vi "FPGA Main.vi"() -> ()   [LabVIEW 2021]
uses:
  <vilib>/Platform/TimedLoop/XDataNode/timing_clust.ctl
  <vilib>/Platform/TimedLoop/XDataNode/nitl_modes.ctl
  <vilib>/Platform/TimedLoop/XDataNode/wakeup.ctl
  <vilib>/rvi/Emulation/niFpgaSctlEmulationGetInTimedLoop.vi
  <vilib>/rvi/Emulation/niFpgaEmulationReportErrorSimple.vi
  <vilib>/rvi/Emulation/niFpgaGetClockAttributes.vi
  <vilib>/rvi/Emulation/niFpgaCriticalErrorInLSC.vi
  <vilib>/rvi/eio/common/nirviEmuTemplateMethod_errors.vi
  <vilib>/rvi/interface/RandomDataEmulation/niFpgaRandomDataHandleErrors.vi
  <vilib>/platform/TimedLoop/XDataNode/XDataNode.xnode
  <vilib>/eio/EIONode/EIONode.xnode
  <vilib>/rvi/DataTransferAndStorage/Container/XNode/niFpgaContainer.xnode
  <vilib>/rvi/interface/RandomDataEmulation/nirviRandomDataFpgaReadWriteTemplate.vi
  <vilib>/Platform/TimedLoop/XDataNode/XDNodeRunTimeDep.lvlib
panel:
  in  "Count(uSec)":u32
  out "Overflow?":bool
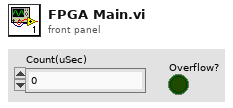
[diagram p1: front panel]
types:
  T1 = typedef "XDNodeRunTimeDep.lvlib/timing_clust.ctl" = cluster{"Expected End [f-1]":u64, "Actual End [f-1]":u64, "Finished Late? [f-1]":bool, "Expected End [i-1]":u64, "Actual End [i-1]":u64, "Finished Late? [i-1]":bool, "Expected Start [i]":u64, "Actual Start [i]":u64, "Expected Start [f]":u64, "Actual Start [f]":u64, "Source Name":string, "Structure Name":string, "Period":i64, "Deadline":i64, "Offset":i64, "Start":i64, "Priority":i32, "Timeout":i32, "Mode":T2, "Wakeup Reason":T3, "Error":errorcluster, "Source Type":string, "Secondary Source Type":string, "Global End Time":u64, "Global Start Time":u64, "Frame Duration":u64, "Iteration Duration":u64, "Assigned CPU":i32, "I/O Scan Engine Mode":u32}
  T2 = typedef "XDNodeRunTimeDep.lvlib/nitl_modes.ctl" = enum32{"No Change", "Process missed periods, maintain original phase", "Discard missed periods, maintain original phase", "Process missed periods, ignore original phase", "Discard missed periods, ignore original phase"}
  T3 = typedef "XDNodeRunTimeDep.lvlib/wakeup.ctl" = enum32{"Normal", "Aborted", "Asynchronous wakeup", "Timing source error", "Timed loop error", "Timeout"}
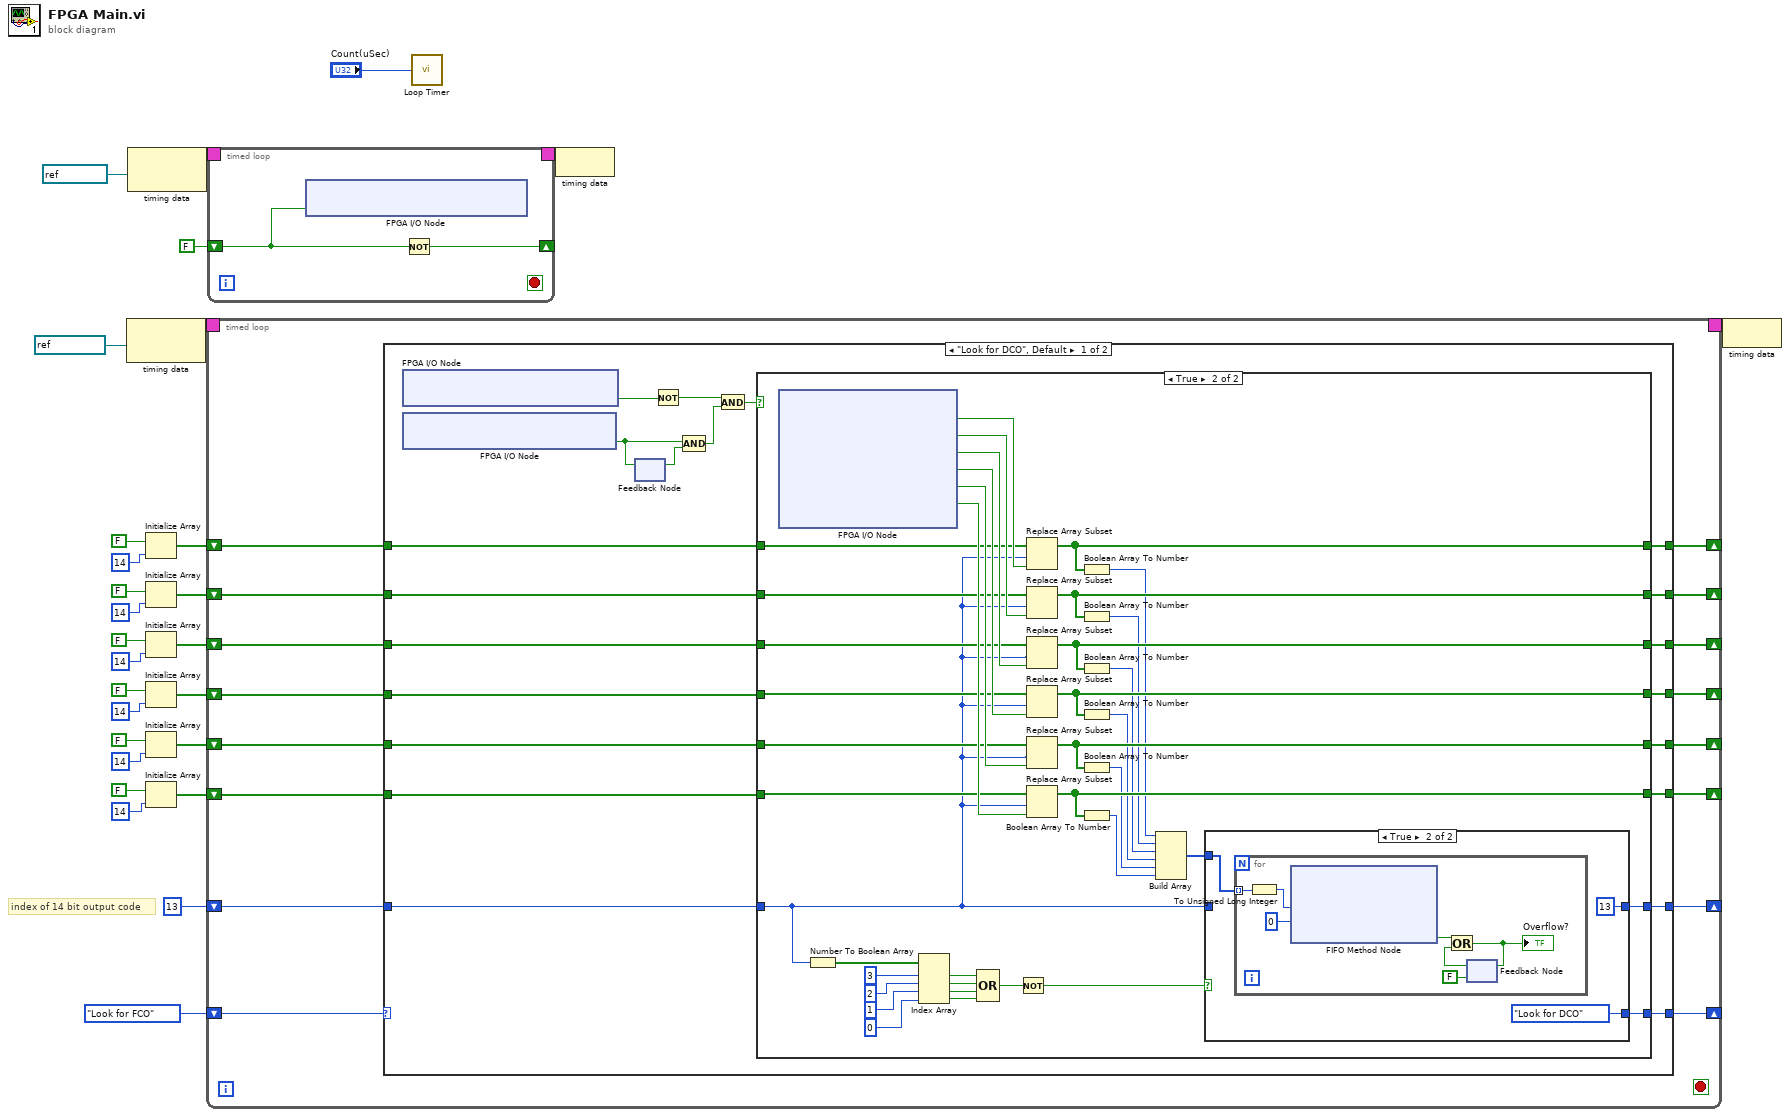
[diagram p0: block diagram]
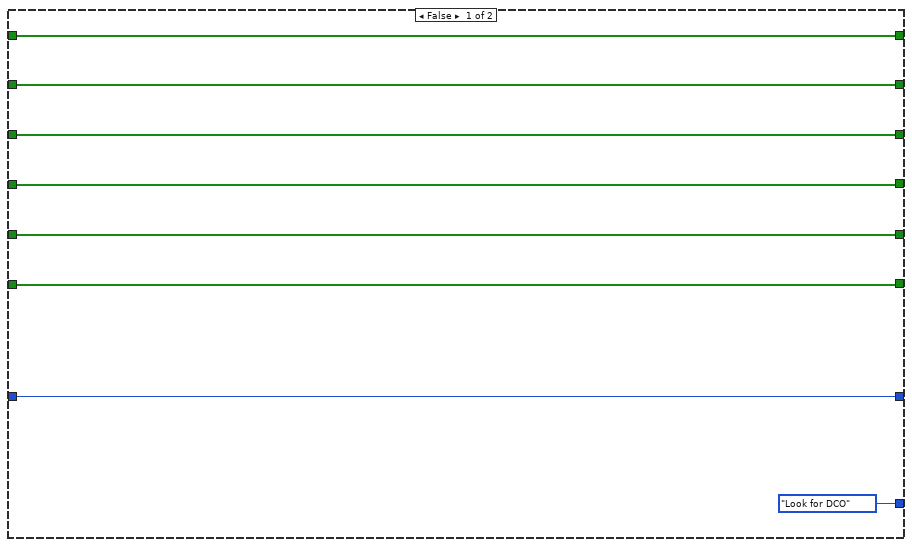
[diagram p2: hidden frame]
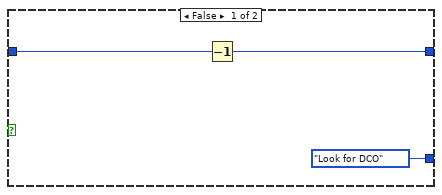
[diagram p3: hidden frame]
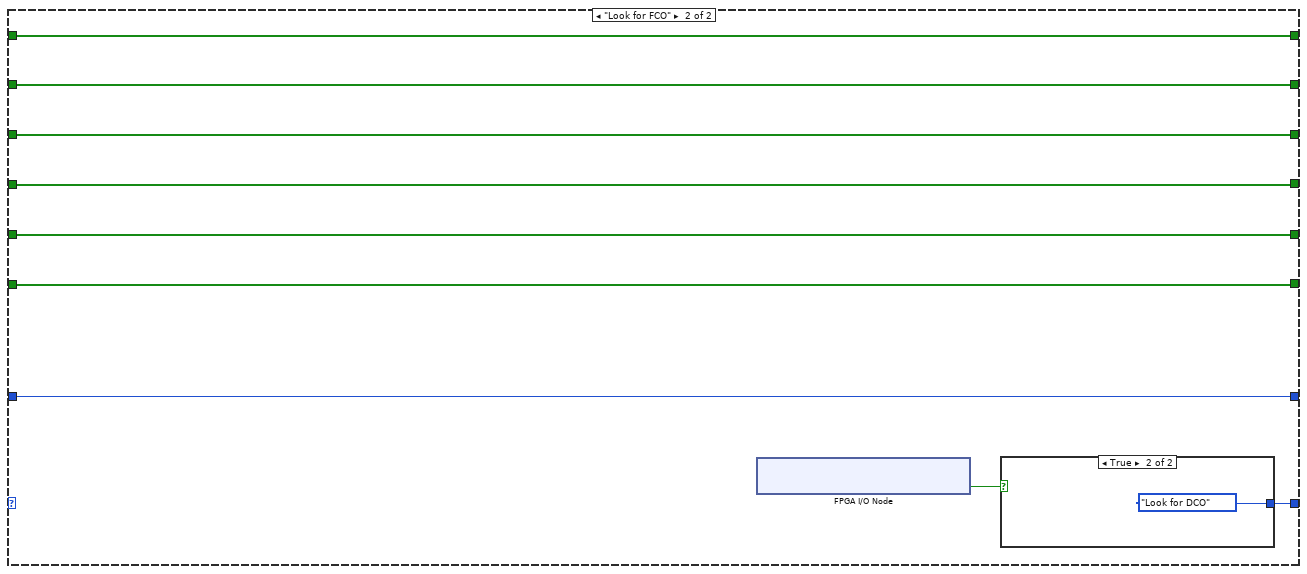
[diagram p4: hidden frame]
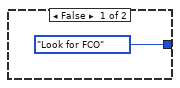
[diagram p5: hidden frame]
diagram:
  # "index of 14 bit output code"
  n1 = node-c288(refnum<k21> "140MHz" ("Source Name")) -> (w24:T1)
  n2 = node-c288(refnum<k21> "20MHz" ("Source Name")) -> (w28:T1)
  n3 = Initialize Array(FALSE, 14) -> (w7:bool[])
  n4 = Initialize Array(FALSE, 14) -> (w6:bool[])
  n5 = Initialize Array(FALSE, 14) -> (w5:bool[])
  n6 = Initialize Array(FALSE, 14) -> (w4:bool[])
  n7 = Initialize Array(FALSE, 14) -> (w3:bool[])
  n8 = Initialize Array(FALSE, 14) -> (w2:bool[])
  n9 = timed-loop {
    timing: w24 -> [_]
    timing-out: [_] -> w23
    shift-right: [w43] -> _
    shift-left: 13 ("index") -> [w44]
    shift-right: [w41] -> _
    shift-left: enum16{"Look for DCO", "Look for FCO"}."Look for FCO" -> [w42]
    shift-right: [w34] -> _
    shift-left: w7 -> [w40]
    shift-right: [w33] -> _
    shift-left: w6 -> [w39]
    shift-right: [w32] -> _
    shift-left: w5 -> [w38]
    shift-right: [w31] -> _
    shift-left: w4 -> [w37]
    shift-right: [w30] -> _
    shift-left: w3 -> [w36]
    shift-right: [w29] -> _
    shift-left: w2 -> [w35]
    stop <- _ stop-if-true
    n10 = case shown="\"Look for DCO\", Default" w42 {
      tunnel: w44 -> [w65 w132]
      tunnel: [w64 w132] -> w43
      tunnel: [w61 w134] -> w41
      tunnel: w40 -> [w56 w131]
      tunnel: w39 -> [w55 w130]
      tunnel: w38 -> [w54 w129]
      tunnel: w37 -> [w53 w128]
      tunnel: w36 -> [w52 w127]
      tunnel: w35 -> [w51 w126]
      tunnel: [w50 w131] -> w34
      tunnel: [w49 w130] -> w33
      tunnel: [w48 w129] -> w32
      tunnel: [w47 w128] -> w31
      tunnel: [w46 w127] -> w30
      tunnel: [w45 w126] -> w29
      frame "Look for DCO", Default {
        n11 = xnode "FPGA I/O Node"() -> ("sbRIO-9651 Socket\\DCO_ADC_in"=w58:bool)  [unwired: 1 in, 1 out]
        n12 = xnode "FPGA I/O Node"() -> ("sbRIO-9651 Socket\\FCO_ADC_in"=w63:bool)  [unwired: 1 in, 1 out]
        n13 = feedback-in #1(w63) -> ()
        n14 = feedback #1() -> (w62:bool)  [unwired: 1 in]
        n15 = Not(x=w58) -> (.not. x?=w57:bool)
        n16 = Compound Arithmetic op=AND(w63, w62) -> (w60:bool)
        n17 = And(x=w57, y=w60) -> (x .and. y?=w59:bool)
        n18 = case shown="True" w59 {
          tunnel: w65 -> [w73 w87]
          tunnel: [w73 w112] -> w64
          tunnel: [enum16{"Look for DCO", "Look for FCO"}."Look for DCO" w100] -> w61
          tunnel: w56 -> [w71 w93]
          tunnel: w55 -> [w70 w92]
          tunnel: w54 -> [w69 w91]
          tunnel: w53 -> [w68 w90]
          tunnel: w52 -> [w67 w89]
          tunnel: w51 -> [w66 w88]
          tunnel: [w71 w86] -> w50
          tunnel: [w70 w85] -> w49
          tunnel: [w69 w84] -> w48
          tunnel: [w68 w83] -> w47
          tunnel: [w67 w82] -> w46
          tunnel: [w66 w81] -> w45
          frame False {
          }
          frame True {
            n19 = xnode "FPGA I/O Node"() -> ("sbRIO-9651 Socket\\DE_in"=w99:bool, "sbRIO-9651 Socket\\DG_in"=w98:bool, "sbRIO-9651 Socket\\DH_in"=w97:bool, "sbRIO-9651 Socket\\DB_in"=w96:bool, "sbRIO-9651 Socket\\DC_in"=w95:bool, "sbRIO-9651 Socket\\DA_in"=w94:bool)  [unwired: 7 in, 8 out]
            n20 = Number To Boolean Array(number=w87) -> (Boolean array=w111:bool[])
            n21 = Index Array(array=w111, index #1=3 ("index"), index #2=2 ("index"), index #3=1 ("index"), index #4=0 ("index")) -> (element #1=w110:bool, element #2=w109:bool, element #3=w108:bool, element #4=w107:bool)
            n22 = Compound Arithmetic op=OR(w110, w109, w108, w107) -> (w106:bool)
            n23 = Not(x=w106) -> (.not. x?=w105:bool)
            n24 = Replace Array Subset(array=w93, new element=w99, index=w87) -> (w86:bool[])
            n25 = Replace Array Subset(array=w92, new element=w98, index=w87) -> (w85:bool[])
            n26 = Replace Array Subset(array=w91, new element=w97, index=w87) -> (w84:bool[])
            n27 = Replace Array Subset(array=w90, new element=w96, index=w87) -> (w83:bool[])
            n28 = Replace Array Subset(array=w89, new element=w95, index=w87) -> (w82:bool[])
            n29 = Replace Array Subset(array=w88, new element=w94, index=w87) -> (w81:bool[])
            n30 = Boolean Array To Number(Boolean array=w86) -> (number=w75:u16)
            n31 = Boolean Array To Number(Boolean array=w85) -> (number=w76:u16)
            n32 = Boolean Array To Number(Boolean array=w84) -> (number=w77:u16)
            n33 = Boolean Array To Number(Boolean array=w83) -> (number=w78:u16)
            n34 = Boolean Array To Number(Boolean array=w82) -> (number=w79:u16)
            n35 = Boolean Array To Number(Boolean array=w81) -> (number=w80:u16)
            n36 = Build Array(w75, w76, w77, w78, w79, w80) -> (w74:u16[])
            n37 = case shown="True" w105 {
              tunnel: w87 -> [w115 _]
              tunnel: [w114 13] -> w112
              tunnel: [enum16{"Look for DCO", "Look for FCO"}."Look for DCO" enum16{"Look for DCO", "Look for FCO"}."Look for DCO"] -> w100
              tunnel: w74 -> [_ w116]
              frame False {
                n38 = Decrement(x=w115) -> (x-1=w114:i32)
              }
              frame True {
                n39 = for {
                  tunnel: w116 -> [w124] mode=indexing
                  n40 = To Unsigned Long Integer(number=w124) -> (unsigned 32bit integer=w123:u32)
                  n41 = xnode ("FIFO Method Node")("Element"=w123, "Timeout"=0) -> ("Timed Out?"=w122:bool)  [unwired: 1 in, 1 out]
                  n42 = feedback #2(FALSE) -> (w121:bool)
                  n43 = Or(x=w122, y=w121) -> (x .or. y?=w120:bool)
                  "Overflow?" <- w120
                  n44 = feedback-in #2(w120) -> ()
                }
              }
            }
          }
        }
      }
      frame "Look for FCO" {
        n45 = xnode "FPGA I/O Node"() -> ("sbRIO-9651 Socket\\FCO_ADC_in"=w133:bool)  [unwired: 1 in, 1 out]
        n46 = case shown="True" w133 {
          tunnel: [enum16{"Look for DCO", "Look for FCO"}."Look for FCO" enum16{"Look for DCO", "Look for FCO"}."Look for DCO"] -> w134
          frame False {
          }
          frame True {
          }
        }
      }
    }
  }
  n47 = timed-loop {
    timing: w28 -> [_]
    timing-out: [_] -> w27
    shift-right: [w140] -> _
    shift-left: FALSE -> [w139]
    stop <- _ stop-if-true
    n48 = xnode "FPGA I/O Node"("sbRIO-9651 Socket\\SCO_ADC_out"=w139) -> ()  [unwired: 1 in, 1 out]
    n49 = Not(x=w139) -> (.not. x?=w140:bool)
  }
  n50 = call "Loop Timer"("Count(uSec)"="Count(uSec)") -> ()  [unwired: 1 out]
  n51 = node-c288(w27) -> ()
  n52 = node-c288(w23) -> ()
